vi "PC Engine.vi"(2 "Error In":errorcluster) -> (0 "Error Out":errorcluster, 1 "InvalidResponses":string)   [LabVIEW 2019]
uses:
  State Ctrl (PC).ctl
  <vilib>/NI/STM/TCP/TCP Connection Info.ctl
  <vilib>/NI/STM/SubVIs/MetaDataElement.ctl
  Event Mode.ctl
  PCsend RTrecv CMD.ctl
  <vilib>/NI/STM/TCP/TCP Read Options.ctl
  RT/RTsend PCrecv CMD.ctl
  TypeDef/ConnSettingCluster.ctl
  <vilib>/NI/STM/TCP/Read Meta Data (TCP Ref).vi
  <vilib>/NI/STM/TCP/Read Message (TCP).vi
  <vilib>/NI/STM/TCP/Read Meta Data (TCP Clst).vi
  <vilib>/NI/STM/TCP/Write Message (TCP).vi
  <vilib>/NI/STM/NI STM.lvlib
panel:
  out "Send Conn Info":T1
  in  "State Control":T3
  in  "Recv Port":u16=5555
  in  "Stop":bool
  out "Connected?":bool
  in  "ConnectAttemptLimit":u32=5
  in  "Send Port":u16=5555
  in  "RIO IP Address":string
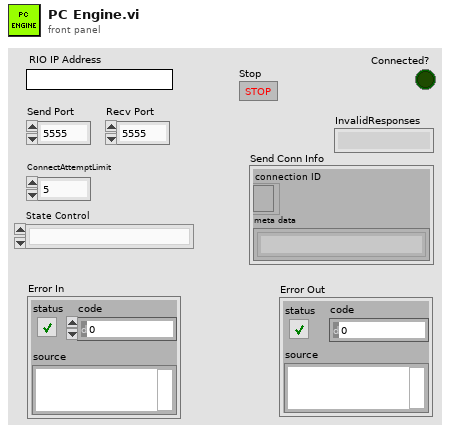
[diagram p1: front panel]
types:
  T1 = typedef "NI STM.lvlib/TCP Connection Info.ctl" = cluster{"connection ID":refnum<k5>, "meta data":T2[]}
  T2 = typedef "NI STM.lvlib/MetaDataElement.ctl" = string
  T3 = typedef "State Ctrl (PC).ctl" = enum16{"", "Send Connect", "Send Connect 2", "Recv Connect", "Recv Connect 2", "No Connection", "Disconnect"}
  T4 = typedef "PCsend RTrecv CMD.ctl" = enum16{"ConnSettings", "Connect", "CMD", "Controller", "PSenable", "ReqCalDate", "Tolerances", "Stable Trigger", "Stop", "VPLimits", "NeedleValve", "SpeedWindow", "FreezeCmdPID", "LoadFPGA", "Tare Pressure"}
  T5 = typedef "Event Mode.ctl" = enum16{"Init", "Get", "Set", "Destroy"}
  T6 = cluster{"Command":string, "Flattened Data":string}
  T7 = typedef "ConnSettingCluster.ctl" = cluster{"ConnectAttemptLimit(5)":u32, "IP Address":string, "Send Port":u16, "Recv Port":u16}
  T8 = typedef "NI STM.lvlib/TCP Read Options.ctl" = cluster{"ignore timeout error":bool, "timeout ms (1000)":i32}
  T9 = typedef "RTsend PCrecv CMD.ctl" = enum16{"Data", "Connected?", "CalFileDate"}
  T10 = cluster{"connection ID":bool, "meta data":bool[]}
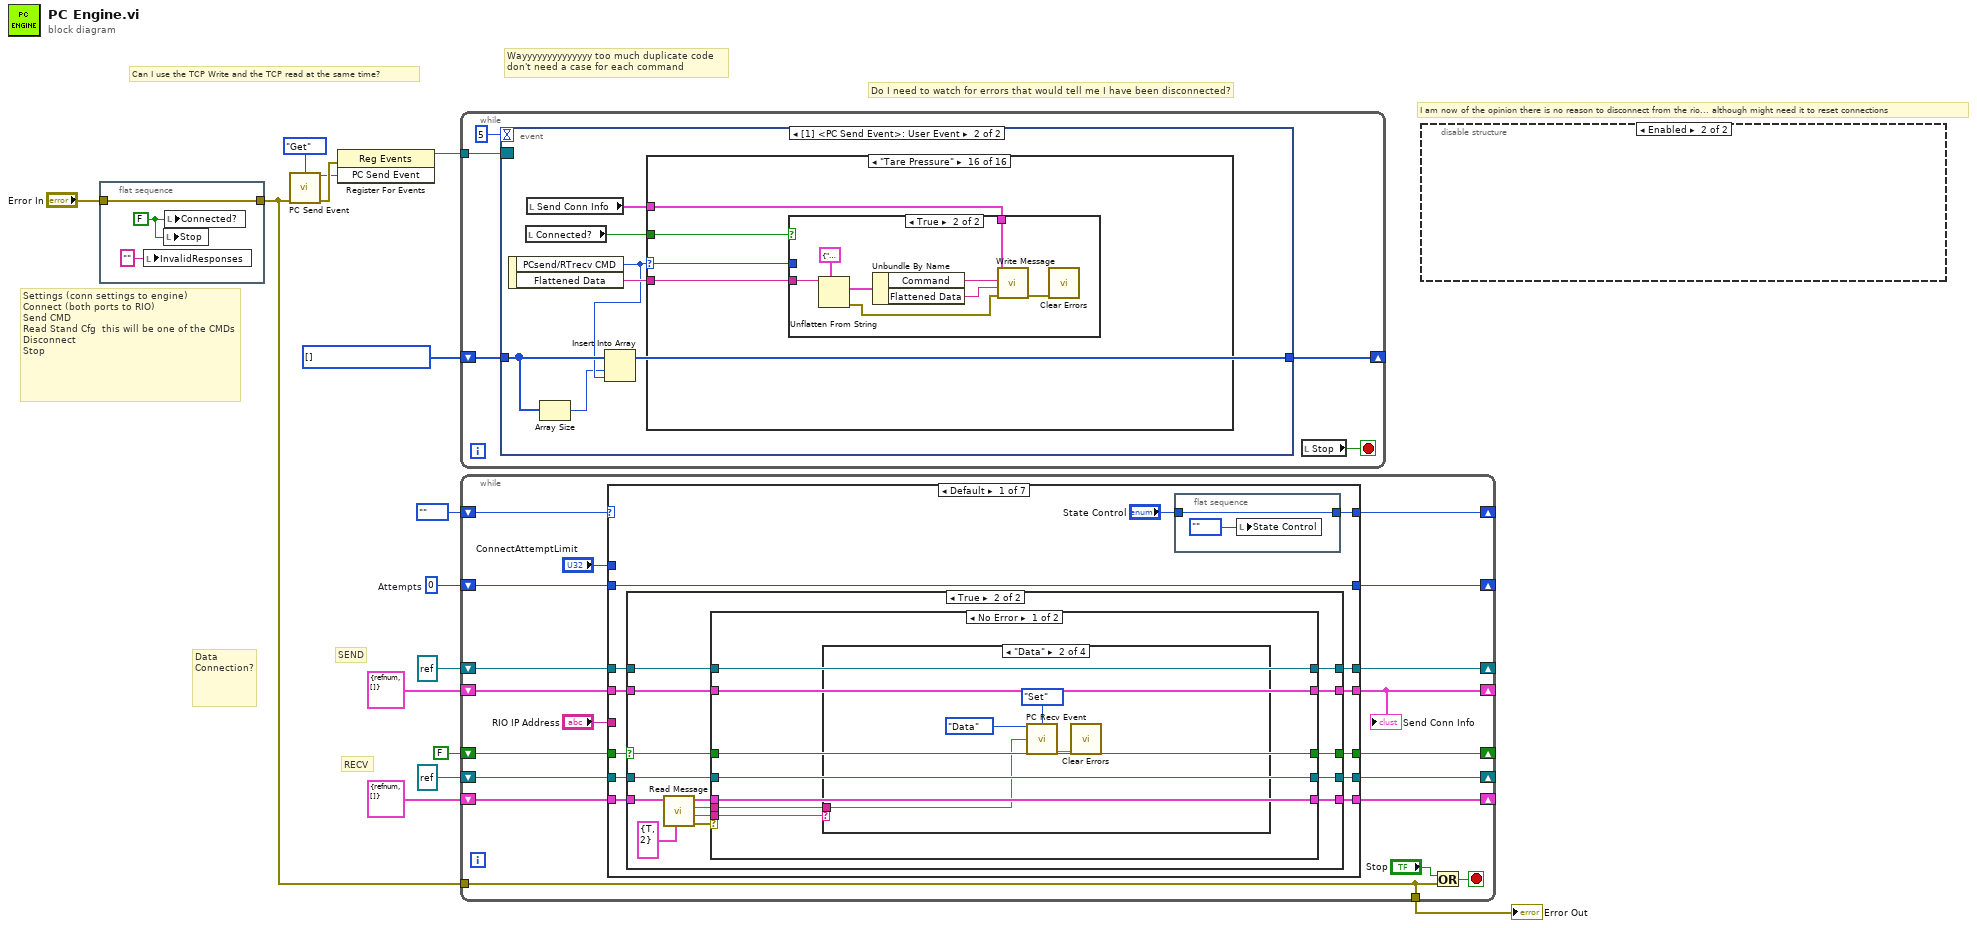
[diagram p0: block diagram]
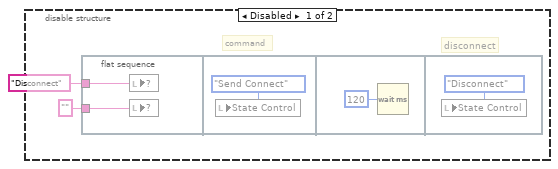
[diagram p2: hidden frame]
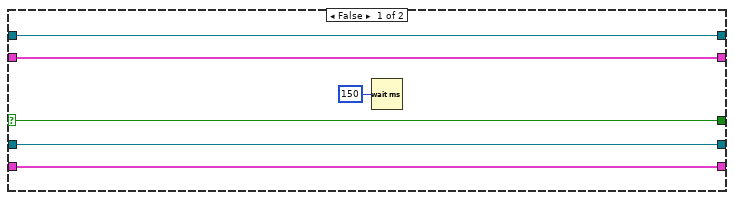
[diagram p3: hidden frame]
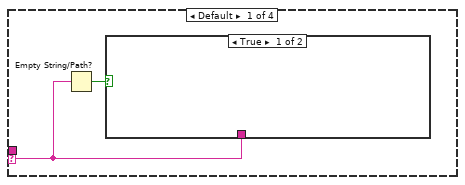
[diagram p4: hidden frame]
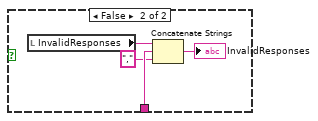
[diagram p5: hidden frame]
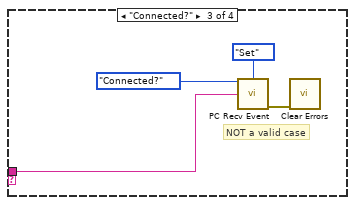
[diagram p6: hidden frame]
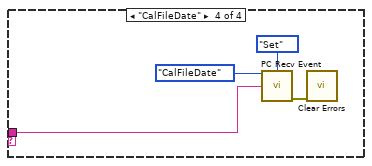
[diagram p7: hidden frame]
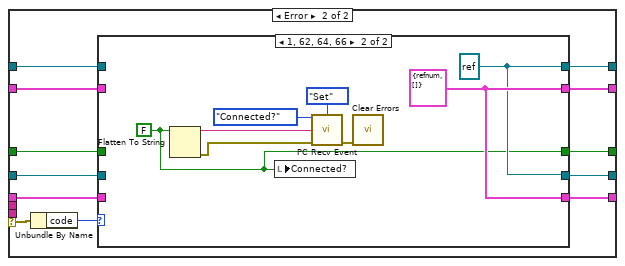
[diagram p8: hidden frame]
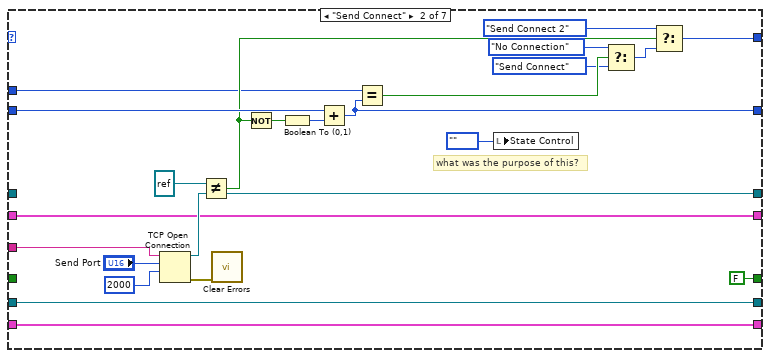
[diagram p10: hidden frame]
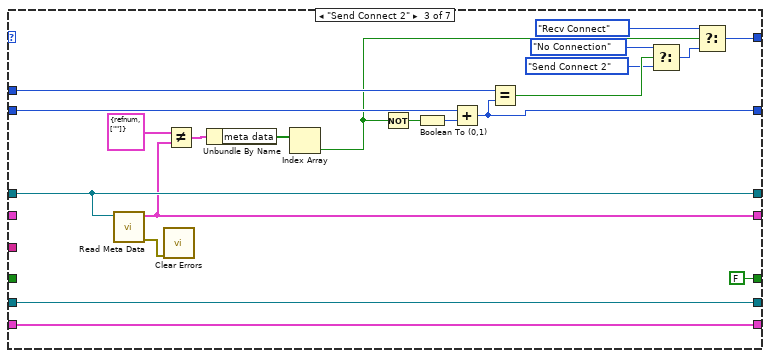
[diagram p11: hidden frame]
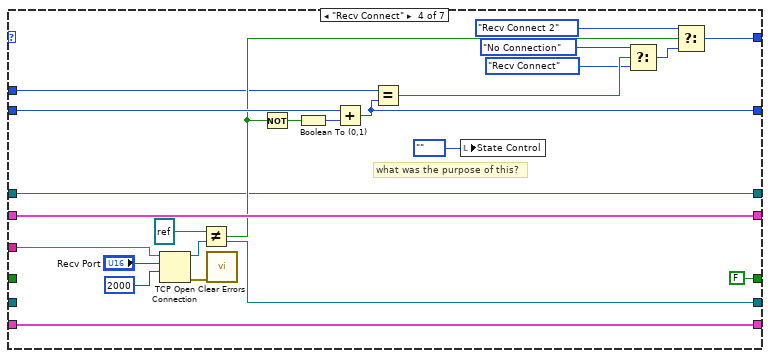
[diagram p12: hidden frame]
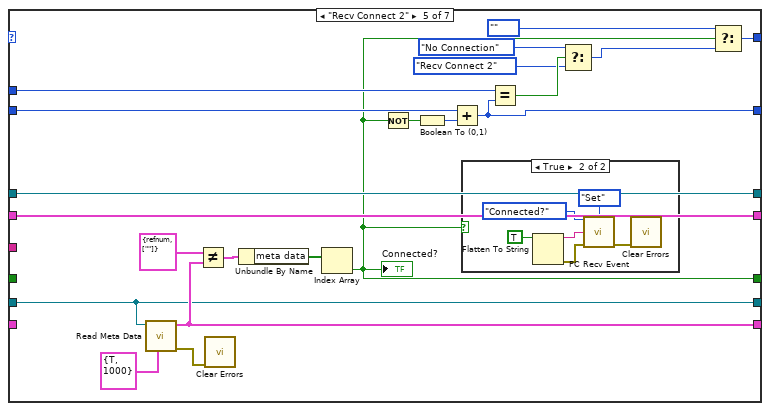
[diagram p13: hidden frame]
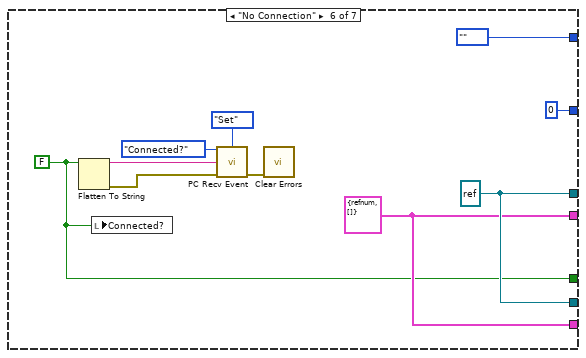
[diagram p15: hidden frame]
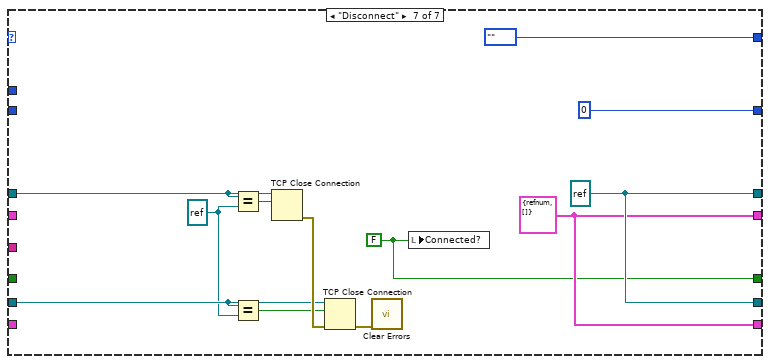
[diagram p16: hidden frame]
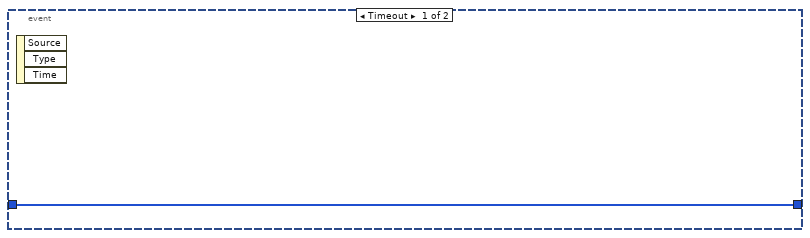
[diagram p17: hidden frame]
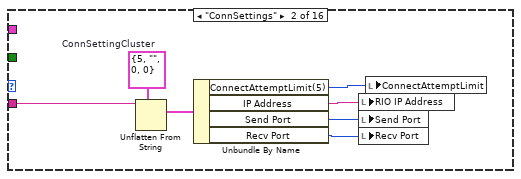
[diagram p19: hidden frame]
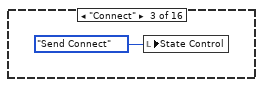
[diagram p20: hidden frame]
diagram:
  w1 = T4[] [] items=["ConnSettings", "Connect", "CMD", "Controller", "PSenable", "ReqCalDate", "Tolerances", "Stable Trigger", "Stop", "VPLimits", "NeedleValve", "SpeedWindow", "FreezeCmdPID", "LoadFPGA", "Tare Pressure"]
  w13 = u32 0  # Attempts
  # "Wayyyyyyyyyyyyyy too much duplicate code\ndon't need a case for each command"
  # "I am now of the opinion there is no reason to disconnect from the rio... although might need it to reset connections"
  # "Do I need to watch for errors that would tell me I have been disconnected?"
  # "RECV"
  # "SEND"
  # "Can I use the TCP Write and the TCP read at the same time?"
  # "Data\nConnection?"
  # "Settings (conn settings to engine)\nConnect (both ports to RIO)\nSend CMD\nRead Stand Cfg  this will be one of the CMDs\nDisconnect\nStop"
  n1 = flat-sequence {
    tunnel: "Error In" -> [w17]
    tunnel: [w17] -> w11
    frame #0 {
      w18 = FALSE ("Connected?")
      n2 = local write "InvalidResponses"("" ("InvalidResponse")) -> ()
      n3 = local write "Stop"(w18) -> ()
      n4 = local write "Connected?"(w18) -> ()
    }
  }
  n5 = call "PC Send Event.vi"("Mode"=Event_Mode."Get", "Error In"=w11) -> ("PC Send Event"=w6:refnum<user-event>, "Error Out"=w8:errorcluster)  [unwired: 12 in]
  n6 = register-events(error in=w8, w6) -> (reference out=w7:refnum<event-registration>)  [unwired: 1 in, 1 out]
  n7 = while {
    tunnel: w7 -> [w21]
    shift-right: [w19] -> _
    shift-left: w1 -> [w20]
    stop <- w23 stop-if-true
    n8 = event shown="[1] <PC Send Event>: User Event" {
      selector: w21 -> [_ _]
      dyn-events: _ -> [_ _]
      timeout: 5 ("evtime") -> [_ _]
      tunnel: w20 -> [w24 w28]
      tunnel: [w24 w25] -> w19
      event Timeout {
        n9 = event-data() -> ()  [unwired: 1 in, 3 out]
      }
      event User Event {
        n10 = event-data() -> ("PCsend/RTrecv CMD"=w27:T4, "Flattened Data"=w31:string)  [unwired: 1 in]
        n11 = local read "Connected?"() -> (w29:bool)
        n12 = local read "Send Conn Info"() -> (w30:T1)
        n13 = Array Size(array=w28) -> (size(s)=w26:i32)
        n14 = Insert Into Array(array=w28, index=w26, new element=w27) -> (w25:T4[])
        n15 = case shown="\"Tare Pressure\"" w27 {
          selector: w27 -> [_ _ _ _ _ _ _ _ _ _ _ _ _ _ _ w162]
          tunnel: w31 -> [_ w33 _ w42 w53 w64 w75 w86 _ w98 w109 w120 w131 w142 w153 w165]
          tunnel: w30 -> [_ _ _ w40 w51 w62 w73 w84 _ w96 w107 w118 w129 w140 w151 w163]
          tunnel: w29 -> [_ _ _ w41 w52 w63 w74 w85 _ w97 w108 w119 w130 w141 w152 w164]
          frame Default {
          }
          frame "ConnSettings" {
            w32 = T7 {"ConnectAttemptLimit(5)"=5, "IP Address"="", "Send Port"=0, "Recv Port"=0}  # ConnSettingCluster
            n16 = Unflatten From String(type=w32, binary string=w33) -> (value=w38:T7)  [unwired: 3 in, 2 out]
            n17 = Unbundle By Name(w38) -> ("ConnectAttemptLimit(5)"=w36:u32, "IP Address"=w35:string, "Send Port"=w37:u16, "Recv Port"=w34:u16)
            n18 = local write "RIO IP Address"(w35) -> ()
            n19 = local write "Send Port"(w37) -> ()
            n20 = local write "Recv Port"(w34) -> ()
            n21 = local write "ConnectAttemptLimit"(w36) -> ()
          }
          frame "Connect" {
            n22 = local write "State Control"(State_Ctrl_(PC)."Send Connect" ("State Control")) -> ()
          }
          frame "CMD" {
            n23 = case shown="True" w41 {
              tunnel: w42 -> [_ w50]
              tunnel: w40 -> [_ w45]
              frame False {
              }
              frame True {
                n24 = Unflatten From String(type=T6 {"Command"="", "Flattened Data"=""} ("cluster"), binary string=w50) -> (value=w49:T6, error out=w43:errorcluster)  [unwired: 3 in, 1 out]
                n25 = Unbundle By Name(w49) -> ("Command"=w46:string, "Flattened Data"=w47:string)
                n26 = call-poly <vilib>:"Write Message.vi"("error in"=w43, "data"=w47, "name"=w46, "connection info in"=w45) -> ("error out"=w44:errorcluster)  [unwired: 6 in, 1 out]
                n27 = call <vilib>:"Clear Errors.vi"("error in (no error)"=w44) -> ()  [unwired: 5 in, 2 out]
              }
            }
          }
          frame "Controller" {
            n28 = case shown="True" w52 {
              tunnel: w53 -> [_ w61]
              tunnel: w51 -> [_ w56]
              frame False {
              }
              frame True {
                n29 = Unflatten From String(type=T6 {"Command"="", "Flattened Data"=""} ("cluster"), binary string=w61) -> (value=w60:T6, error out=w54:errorcluster)  [unwired: 3 in, 1 out]
                n30 = Unbundle By Name(w60) -> ("Command"=w57:string, "Flattened Data"=w58:string)
                n31 = call-poly <vilib>:"Write Message.vi"("error in"=w54, "data"=w58, "name"=w57, "connection info in"=w56) -> ("error out"=w55:errorcluster)  [unwired: 6 in, 1 out]
                n32 = call <vilib>:"Clear Errors.vi"("error in (no error)"=w55) -> ()  [unwired: 5 in, 2 out]
              }
            }
          }
          frame "PSenable" {
            n33 = case shown="True" w63 {
              tunnel: w64 -> [_ w72]
              tunnel: w62 -> [_ w67]
              frame False {
              }
              frame True {
                n34 = Unflatten From String(type=T6 {"Command"="", "Flattened Data"=""} ("cluster"), binary string=w72) -> (value=w71:T6, error out=w65:errorcluster)  [unwired: 3 in, 1 out]
                n35 = Unbundle By Name(w71) -> ("Command"=w68:string, "Flattened Data"=w69:string)
                n36 = call-poly <vilib>:"Write Message.vi"("error in"=w65, "data"=w69, "name"=w68, "connection info in"=w67) -> ("error out"=w66:errorcluster)  [unwired: 6 in, 1 out]
                n37 = call <vilib>:"Clear Errors.vi"("error in (no error)"=w66) -> ()  [unwired: 5 in, 2 out]
              }
            }
          }
          frame "ReqCalDate" {
            n38 = case shown="True" w74 {
              tunnel: w75 -> [_ w83]
              tunnel: w73 -> [_ w78]
              frame False {
              }
              frame True {
                n39 = Unflatten From String(type=T6 {"Command"="", "Flattened Data"=""} ("cluster"), binary string=w83) -> (value=w82:T6, error out=w76:errorcluster)  [unwired: 3 in, 1 out]
                n40 = Unbundle By Name(w82) -> ("Command"=w79:string, "Flattened Data"=w80:string)
                n41 = call-poly <vilib>:"Write Message.vi"("error in"=w76, "data"=w80, "name"=w79, "connection info in"=w78) -> ("error out"=w77:errorcluster)  [unwired: 6 in, 1 out]
                n42 = call <vilib>:"Clear Errors.vi"("error in (no error)"=w77) -> ()  [unwired: 5 in, 2 out]
              }
            }
          }
          frame "Tolerances" {
            n43 = case shown="True" w85 {
              tunnel: w86 -> [_ w94]
              tunnel: w84 -> [_ w89]
              frame False {
              }
              frame True {
                n44 = Unflatten From String(type=T6 {"Command"="", "Flattened Data"=""} ("cluster"), binary string=w94) -> (value=w93:T6, error out=w87:errorcluster)  [unwired: 3 in, 1 out]
                n45 = Unbundle By Name(w93) -> ("Command"=w90:string, "Flattened Data"=w91:string)
                n46 = call-poly <vilib>:"Write Message.vi"("error in"=w87, "data"=w91, "name"=w90, "connection info in"=w89) -> ("error out"=w88:errorcluster)  [unwired: 6 in, 1 out]
                n47 = call <vilib>:"Clear Errors.vi"("error in (no error)"=w88) -> ()  [unwired: 5 in, 2 out]
              }
            }
          }
          frame "Stop" {
            n48 = local write "Stop"(TRUE ("Stop")) -> ()
          }
          frame "VPLimits" {
            n49 = case shown="True" w97 {
              tunnel: w98 -> [_ w106]
              tunnel: w96 -> [_ w101]
              frame False {
              }
              frame True {
                n50 = Unflatten From String(type=T6 {"Command"="", "Flattened Data"=""} ("cluster"), binary string=w106) -> (value=w105:T6, error out=w99:errorcluster)  [unwired: 3 in, 1 out]
                n51 = Unbundle By Name(w105) -> ("Command"=w102:string, "Flattened Data"=w103:string)
                n52 = call-poly <vilib>:"Write Message.vi"("error in"=w99, "data"=w103, "name"=w102, "connection info in"=w101) -> ("error out"=w100:errorcluster)  [unwired: 6 in, 1 out]
                n53 = call <vilib>:"Clear Errors.vi"("error in (no error)"=w100) -> ()  [unwired: 5 in, 2 out]
              }
            }
          }
          frame "NeedleValve" {
            n54 = case shown="True" w108 {
              tunnel: w109 -> [_ w117]
              tunnel: w107 -> [_ w112]
              frame False {
              }
              frame True {
                n55 = Unflatten From String(type=T6 {"Command"="", "Flattened Data"=""} ("cluster"), binary string=w117) -> (value=w116:T6, error out=w110:errorcluster)  [unwired: 3 in, 1 out]
                n56 = Unbundle By Name(w116) -> ("Command"=w113:string, "Flattened Data"=w114:string)
                n57 = call-poly <vilib>:"Write Message.vi"("error in"=w110, "data"=w114, "name"=w113, "connection info in"=w112) -> ("error out"=w111:errorcluster)  [unwired: 6 in, 1 out]
                n58 = call <vilib>:"Clear Errors.vi"("error in (no error)"=w111) -> ()  [unwired: 5 in, 2 out]
              }
            }
          }
          frame "SpeedWindow" {
            n59 = case shown="True" w119 {
              tunnel: w120 -> [_ w128]
              tunnel: w118 -> [_ w123]
              frame False {
              }
              frame True {
                n60 = Unflatten From String(type=T6 {"Command"="", "Flattened Data"=""} ("cluster"), binary string=w128) -> (value=w127:T6, error out=w121:errorcluster)  [unwired: 3 in, 1 out]
                n61 = Unbundle By Name(w127) -> ("Command"=w124:string, "Flattened Data"=w125:string)
                n62 = call-poly <vilib>:"Write Message.vi"("error in"=w121, "data"=w125, "name"=w124, "connection info in"=w123) -> ("error out"=w122:errorcluster)  [unwired: 6 in, 1 out]
                n63 = call <vilib>:"Clear Errors.vi"("error in (no error)"=w122) -> ()  [unwired: 5 in, 2 out]
              }
            }
          }
          frame "FreezeCmdPID" {
            n64 = case shown="True" w130 {
              tunnel: w131 -> [_ w139]
              tunnel: w129 -> [_ w134]
              frame False {
              }
              frame True {
                n65 = Unflatten From String(type=T6 {"Command"="", "Flattened Data"=""} ("cluster"), binary string=w139) -> (value=w138:T6, error out=w132:errorcluster)  [unwired: 3 in, 1 out]
                n66 = Unbundle By Name(w138) -> ("Command"=w135:string, "Flattened Data"=w136:string)
                n67 = call-poly <vilib>:"Write Message.vi"("error in"=w132, "data"=w136, "name"=w135, "connection info in"=w134) -> ("error out"=w133:errorcluster)  [unwired: 6 in, 1 out]
                n68 = call <vilib>:"Clear Errors.vi"("error in (no error)"=w133) -> ()  [unwired: 5 in, 2 out]
              }
            }
          }
          frame "LoadFPGA" {
            n69 = case shown="True" w141 {
              tunnel: w142 -> [_ w150]
              tunnel: w140 -> [_ w145]
              frame False {
              }
              frame True {
                n70 = Unflatten From String(type=T6 {"Command"="", "Flattened Data"=""} ("cluster"), binary string=w150) -> (value=w149:T6, error out=w143:errorcluster)  [unwired: 3 in, 1 out]
                n71 = Unbundle By Name(w149) -> ("Command"=w146:string, "Flattened Data"=w147:string)
                n72 = call-poly <vilib>:"Write Message.vi"("error in"=w143, "data"=w147, "name"=w146, "connection info in"=w145) -> ("error out"=w144:errorcluster)  [unwired: 6 in, 1 out]
                n73 = call <vilib>:"Clear Errors.vi"("error in (no error)"=w144) -> ()  [unwired: 5 in, 2 out]
              }
            }
          }
          frame "Stable Trigger" {
            n74 = case shown="True" w152 {
              tunnel: w153 -> [_ w161]
              tunnel: w151 -> [_ w156]
              frame False {
              }
              frame True {
                n75 = Unflatten From String(type=T6 {"Command"="", "Flattened Data"=""} ("cluster"), binary string=w161) -> (value=w160:T6, error out=w154:errorcluster)  [unwired: 3 in, 1 out]
                n76 = Unbundle By Name(w160) -> ("Command"=w157:string, "Flattened Data"=w158:string)
                n77 = call-poly <vilib>:"Write Message.vi"("error in"=w154, "data"=w158, "name"=w157, "connection info in"=w156) -> ("error out"=w155:errorcluster)  [unwired: 6 in, 1 out]
                n78 = call <vilib>:"Clear Errors.vi"("error in (no error)"=w155) -> ()  [unwired: 5 in, 2 out]
              }
            }
          }
          frame "Tare Pressure" {
            n79 = case shown="True" w164 {
              tunnel: w165 -> [_ w173]
              tunnel: w163 -> [_ w170]
              tunnel: w162 -> [_ _]
              frame False {
              }
              frame True {
                n80 = Unflatten From String(type=T6 {"Command"="", "Flattened Data"=""} ("cluster"), binary string=w173) -> (value=w172:T6, error out=w168:errorcluster)  [unwired: 3 in, 1 out]
                n81 = Unbundle By Name(w172) -> ("Command"=w166:string, "Flattened Data"=w167:string)
                n82 = call-poly <vilib>:"Write Message.vi"("error in"=w168, "data"=w167, "name"=w166, "connection info in"=w170) -> ("error out"=w169:errorcluster)  [unwired: 6 in, 1 out]
                n83 = call <vilib>:"Clear Errors.vi"("error in (no error)"=w169) -> ()  [unwired: 5 in, 2 out]
              }
            }
          }
        }
      }
    }
    n84 = local read "Stop"() -> (w23:bool)
  }
  n85 = while {
    shift-right: [w187] -> _
    shift-left: refnum<k5> refnum ("connection ID") -> [w190]
    shift-right: [w188] -> _
    shift-left: T1 {"connection ID"=refnum, "meta data"=[]} ("connection info out") -> [w189]
    shift-right: [w191] -> _
    shift-left: State_Ctrl_(PC)."" ("State Control") -> [w192]
    shift-right: [w185] -> _
    shift-left: w13 -> [w186]
    tunnel: w11 -> [w174]
    shift-right: [w178] -> _
    shift-left: refnum<k5> refnum ("connection ID") -> [w180]
    shift-right: [w177] -> _
    shift-left: T1 {"connection ID"=refnum, "meta data"=[]} ("connection info out") -> [w179]
    shift-right: [w175] -> _
    shift-left: FALSE -> [w176]
    tunnel: [w174] -> w2
    stop <- w183 stop-if-true
    n86 = case shown="Default" w192 {
      tunnel: [w205 w301 w319 w345 w363 State_Ctrl_(PC)."" ("State Control") State_Ctrl_(PC)."" ("State Control")] -> w191
      tunnel: w190 -> [w200 _ w320 w327 w364 _ w389]
      tunnel: w189 -> [w201 w296 _ w342 w351 _ _]
      tunnel: [w197 w296 w303 w342 w351 w377 w391] -> w188
      tunnel: [w198 w297 w320 w327 w364 w378 w392] -> w187
      tunnel: w186 -> [w193 w295 w315 w341 w359 _ _]
      tunnel: [w193 w291 w314 w337 w358 u32 0 ("Attempts") u32 0 ("Attempts")] -> w185
      tunnel: "ConnectAttemptLimit" -> [_ w288 w312 w334 w356 _ _]
      tunnel: "RIO IP Address" -> [_ w283 _ w329 _ _ _]
      tunnel: w180 -> [w199 w282 w308 _ w350 _ w386]
      tunnel: w179 -> [w202 w281 w307 w325 _ _ _]
      tunnel: [w195 w282 w308 w326 w350 w378 w392] -> w178
      tunnel: [w194 w281 w307 w325 w352 w377 w391] -> w177
      tunnel: w176 -> [w203 _ _ _ _ _ _]
      tunnel: [w196 FALSE ("Meta Element") FALSE ("Meta Element") FALSE ("Meta Element") w347 w376 w384] -> w175
      frame Default {
        n87 = case shown="True" w203 {
          selector: w203 -> [w209 w220]
          tunnel: w202 -> [w207 w225]
          tunnel: w201 -> [w210 w221]
          tunnel: w200 -> [w211 w219]
          tunnel: w199 -> [w208 w222]
          tunnel: [w211 w217] -> w198
          tunnel: [w210 w215] -> w197
          tunnel: [w209 w218] -> w196
          tunnel: [w208 w216] -> w195
          tunnel: [w207 w214] -> w194
          frame False {
            n88 = Wait (ms)(milliseconds to wait=u32 150) -> ()  [unwired: 1 out]
          }
          frame True {
            n89 = call-poly <vilib>:"Read Message.vi"("options"=T8 {"ignore timeout error"=TRUE, "timeout ms (1000)"=2}, "connection info in"=w225) -> ("error out"=w224:errorcluster, "name"=w213:T2, "data string"=w212:string, "connection info out"=w223:T1)  [unwired: 4 in, 2 out]
            n90 = case shown="No Error" w224 {
              selector: w224 -> [_ w263]
              tunnel: w223 -> [w229 w261]
              tunnel: w222 -> [w230 w260]
              tunnel: w221 -> [w232 w258]
              tunnel: w220 -> [w231 w259]
              tunnel: w219 -> [w233 w257]
              tunnel: [w231 w254] -> w218
              tunnel: [w233 w256] -> w217
              tunnel: [w230 w253] -> w216
              tunnel: [w232 w255] -> w215
              tunnel: [w229 w252] -> w214
              tunnel: w213 -> [w228 _]
              tunnel: w212 -> [w227 _]
              frame No Error {
                n91 = case shown="\"Data\"" w228 {
                  selector: w228 -> [w235 _ _ _]
                  tunnel: w227 -> [_ w243 w246 w250]
                  frame Default {
                    n92 = Empty String/Path?(string/path=w235) -> (empty?=w234:bool)
                    n93 = case shown="True" w234 {
                      tunnel: w235 -> [_ w238]
                      frame True {
                      }
                      frame False {
                        n94 = local read "InvalidResponses"() -> (w239:string)
                        n95 = Concatenate Strings(w239, w238, "," ("string")) -> (→"InvalidResponses":string)
                      }
                    }
                  }
                  frame "Data" {
                    n96 = call "PC Recv Event.vi"("RTsend/PCrecv CMD"=RTsend_PCrecv_CMD."Data", "Mode"=Event_Mode."Set", "Flattened Data"=w243) -> ("Error Out"=w241:errorcluster)  [unwired: 11 in, 1 out]
                    n97 = call <vilib>:"Clear Errors.vi"("error in (no error)"=w241) -> ()  [unwired: 5 in, 2 out]
                  }
                  frame "Connected?" {
                    # "NOT a valid case"
                    n98 = call "PC Recv Event.vi"("RTsend/PCrecv CMD"=RTsend_PCrecv_CMD."Connected?", "Mode"=Event_Mode."Set", "Flattened Data"=w246) -> ("Error Out"=w245:errorcluster)  [unwired: 11 in, 1 out]
                    n99 = call <vilib>:"Clear Errors.vi"("error in (no error)"=w245) -> ()  [unwired: 5 in, 2 out]
                  }
                  frame "CalFileDate" {
                    n100 = call "PC Recv Event.vi"("RTsend/PCrecv CMD"=RTsend_PCrecv_CMD."CalFileDate", "Mode"=Event_Mode."Set", "Flattened Data"=w250) -> ("Error Out"=w249:errorcluster)  [unwired: 11 in, 1 out]
                    n101 = call <vilib>:"Clear Errors.vi"("error in (no error)"=w249) -> ()  [unwired: 5 in, 2 out]
                  }
                }
              }
              frame Error {
                n102 = Unbundle By Name(w263) -> ("code"=w262:i32)
                n103 = case shown="1, 62, 64, 66" w262 {
                  tunnel: w261 -> [w264 _]
                  tunnel: w260 -> [w265 _]
                  tunnel: w259 -> [w266 _]
                  tunnel: w258 -> [w267 _]
                  tunnel: w257 -> [w268 _]
                  tunnel: [w268 w275] -> w256
                  tunnel: [w267 w276] -> w255
                  tunnel: [w266 w272] -> w254
                  tunnel: [w265 w275] -> w253
                  tunnel: [w264 w276] -> w252
                  frame Default {
                  }
                  frame 1, 62, 64, 66 {
                    w272 = FALSE ("Connected?")
                    w276 = T1 {"connection ID"=refnum, "meta data"=[]} ("connection info out")
                    w275 = refnum<k5> refnum ("connection ID")
                    n104 = Flatten To String(anything=w272) -> (data string=w273:string, error out=w271:errorcluster)  [unwired: 3 in, 1 out]
                    n105 = local write "Connected?"(w272) -> ()
                    n106 = call "PC Recv Event.vi"("RTsend/PCrecv CMD"=RTsend_PCrecv_CMD."Connected?", "Mode"=Event_Mode."Set", "Flattened Data"=w273, "Error In"=w271) -> ("Error Out"=w270:errorcluster)  [unwired: 10 in, 1 out]
                    n107 = call <vilib>:"Clear Errors.vi"("error in (no error)"=w270) -> ()  [unwired: 5 in, 2 out]
                  }
                }
              }
            }
          }
        }
        n108 = flat-sequence {
          tunnel: "State Control" -> [w278]
          tunnel: [w278] -> w205
          frame #0 {
            n109 = local write "State Control"(State_Ctrl_(PC)."" ("State Control")) -> ()
          }
        }
      }
      frame "Send Connect" {
        # "what was the purpose of this?"
        n110 = TCP Open Connection(address=w283, remote port or service name="Send Port", timeout ms (60000)=2000) -> (connection ID=w297:refnum<k5>, error out=w279:errorcluster)  [unwired: 2 in]
        n111 = Not Equal?(x=refnum<k5> refnum ("connection ID"), y=w297) -> (x != y?=w294:bool)
        n112 = call <vilib>:"Clear Errors.vi"("error in (no error)"=w279) -> ()  [unwired: 5 in, 2 out]
        n113 = Not(x=w294) -> (.not. x?=w293:bool)
        n114 = Boolean To (0,1)(Boolean=w293) -> (0, 1=w292:i16)
        n115 = Add(x=w295, y=w292) -> (x+y=w291:u32)
        n116 = Equal?(x=w288, y=w291) -> (x = y?=w290:bool)
        n117 = local write "State Control"(State_Ctrl_(PC)."" ("State Control")) -> ()
        n118 = Select(t=State_Ctrl_(PC)."No Connection" ("State Control"), s=w290, f=State_Ctrl_(PC)."Send Connect" ("State Control")) -> (s? t:f=w289:T3)
        n119 = Select(t=State_Ctrl_(PC)."Send Connect 2" ("State Control"), s=w294, f=w289) -> (s? t:f=w301:T3)
      }
      frame "Send Connect 2" {
        n120 = call-poly <vilib>:"Read Meta Data.vi"("connection ID"=w320) -> ("error out"=w304:errorcluster, "connection info out"=w303:T1)  [unwired: 8 in, 1 out]
        n121 = call <vilib>:"Clear Errors.vi"("error in (no error)"=w304) -> ()  [unwired: 5 in, 2 out]
        n122 = Not Equal?(x=T1 {"connection ID"=refnum, "meta data"=[""]} ("connection info out"), y=w303) -> (x != y?=w322:T10)
        n123 = Unbundle By Name(w322) -> ("meta data"=w311:bool[])
        n124 = Index Array(array=w311) -> (element=w302:bool)  [unwired: 1 in]
        n125 = Not(x=w302) -> (.not. x?=w317:bool)
        n126 = Boolean To (0,1)(Boolean=w317) -> (0, 1=w316:i16)
        n127 = Add(x=w315, y=w316) -> (x+y=w314:u32)
        n128 = Equal?(x=w312, y=w314) -> (x = y?=w313:bool)
        n129 = Select(t=State_Ctrl_(PC)."No Connection" ("State Control"), s=w313, f=State_Ctrl_(PC)."Send Connect 2" ("State Control")) -> (s? t:f=w318:T3)
        n130 = Select(t=State_Ctrl_(PC)."Recv Connect" ("State Control"), s=w302, f=w318) -> (s? t:f=w319:T3)
      }
      frame "Recv Connect" {
        # "what was the purpose of this?"
        n131 = TCP Open Connection(address=w329, remote port or service name="Recv Port", timeout ms (60000)=2000) -> (connection ID=w326:refnum<k5>, error out=w323:errorcluster)  [unwired: 2 in]
        n132 = Not Equal?(x=refnum<k5> refnum ("connection ID"), y=w326) -> (x != y?=w340:bool)
        n133 = call <vilib>:"Clear Errors.vi"("error in (no error)"=w323) -> ()  [unwired: 5 in, 2 out]
        n134 = Not(x=w340) -> (.not. x?=w339:bool)
        n135 = Boolean To (0,1)(Boolean=w339) -> (0, 1=w338:i16)
        n136 = Add(x=w341, y=w338) -> (x+y=w337:u32)
        n137 = Equal?(x=w334, y=w337) -> (x = y?=w336:bool)
        n138 = local write "State Control"(State_Ctrl_(PC)."" ("State Control")) -> ()
        n139 = Select(t=State_Ctrl_(PC)."No Connection" ("State Control"), s=w336, f=State_Ctrl_(PC)."Recv Connect" ("State Control")) -> (s? t:f=w335:T3)
        n140 = Select(t=State_Ctrl_(PC)."Recv Connect 2" ("State Control"), s=w340, f=w335) -> (s? t:f=w345:T3)
      }
      frame "Recv Connect 2" {
        n141 = call-poly <vilib>:"Read Meta Data.vi"("options"=T8 {"ignore timeout error"=TRUE, "timeout ms (1000)"=1000}, "connection ID"=w350) -> ("error out"=w349:errorcluster, "connection info out"=w352:T1)  [unwired: 7 in, 1 out]
        n142 = Not Equal?(x=T1 {"connection ID"=refnum, "meta data"=[""]} ("connection info out"), y=w352) -> (x != y?=w366:T10)
        n143 = call <vilib>:"Clear Errors.vi"("error in (no error)"=w349) -> ()  [unwired: 5 in, 2 out]
        n144 = Unbundle By Name(w366) -> ("meta data"=w355:bool[])
        n145 = Index Array(array=w355) -> (element=w347:bool)  [unwired: 1 in]
        "Connected?" <- w347
        n146 = Not(x=w347) -> (.not. x?=w361:bool)
        n147 = Boolean To (0,1)(Boolean=w361) -> (0, 1=w360:i16)
        n148 = Add(x=w359, y=w360) -> (x+y=w358:u32)
        n149 = case shown="True" w347 {
          frame False {
          }
          frame True {
            n150 = Flatten To String(anything=TRUE) -> (data string=w370:string, error out=w369:errorcluster)  [unwired: 3 in, 1 out]
            n151 = call "PC Recv Event.vi"("RTsend/PCrecv CMD"=RTsend_PCrecv_CMD."Connected?", "Mode"=Event_Mode."Set", "Flattened Data"=w370, "Error In"=w369) -> ("Error Out"=w368:errorcluster)  [unwired: 10 in, 1 out]
            n152 = call <vilib>:"Clear Errors.vi"("error in (no error)"=w368) -> ()  [unwired: 5 in, 2 out]
          }
        }
        n153 = Equal?(x=w356, y=w358) -> (x = y?=w357:bool)
        n154 = Select(t=State_Ctrl_(PC)."No Connection" ("State Control"), s=w357, f=State_Ctrl_(PC)."Recv Connect 2" ("State Control")) -> (s? t:f=w362:T3)
        n155 = Select(t=State_Ctrl_(PC)."" ("State Control"), s=w347, f=w362) -> (s? t:f=w363:T3)
      }
      frame "No Connection" {
        w376 = FALSE
        w377 = T1 {"connection ID"=refnum, "meta data"=[]} ("connection info out")
        w378 = refnum<k5> refnum ("connection ID")
        n156 = Flatten To String(anything=w376) -> (data string=w380:string, error out=w375:errorcluster)  [unwired: 3 in, 1 out]
        n157 = local write "Connected?"(w376) -> ()
        n158 = call "PC Recv Event.vi"("RTsend/PCrecv CMD"=RTsend_PCrecv_CMD."Connected?", "Mode"=Event_Mode."Set", "Flattened Data"=w380, "Error In"=w375) -> ("Error Out"=w374:errorcluster)  [unwired: 10 in, 1 out]
        n159 = call <vilib>:"Clear Errors.vi"("error in (no error)"=w374) -> ()  [unwired: 5 in, 2 out]
      }
      frame "Disconnect" {
        w384 = FALSE ("Connected?")
        w385 = refnum<k5> refnum ("connection ID")
        w391 = T1 {"connection ID"=refnum, "meta data"=[]} ("connection info out")
        w392 = refnum<k5> refnum ("connection ID")
        n160 = Equal?(x=w389, y=w385) -> (x = y?=w388:bool)
        n161 = Equal?(x=w386, y=w385) -> (x = y?=w387:bool)
        n162 = TCP Close Connection(connection ID=w389, abort (F)=w388) -> (error out=w390:errorcluster)  [unwired: 1 in, 1 out]
        n163 = TCP Close Connection(connection ID=w386, abort (F)=w387, error in (no error)=w390) -> (error out=w383:errorcluster)  [unwired: 1 out]
        n164 = call <vilib>:"Clear Errors.vi"("error in (no error)"=w383) -> ()  [unwired: 5 in, 2 out]
        n165 = local write "Connected?"(w384) -> ()
      }
    }
    "Send Conn Info" <- w188
    n166 = Or(x="Stop", y=w174) -> (x .or. y?=w183:bool)
  }
  "Error Out" <- w2
  n167 = disable-structure shown="Enabled" {
    frame Disabled {
      # "disconnect"
      # "command"
      n168 = flat-sequence {
        tunnel: "" ("Flattened Data") -> [w398]
        tunnel: "Disconnect" ("Command") -> [w397]
        frame #0 {
          n169 = local write item#-1(w397) -> ()
          n170 = local write item#-1(w398) -> ()
        }
        frame #1 {
          n171 = local write "State Control"(State_Ctrl_(PC)."Send Connect" ("State Control")) -> ()
        }
        frame #2 {
          n172 = Wait (ms)(milliseconds to wait=u32 120) -> ()  [unwired: 1 out]
        }
        frame #3 {
          n173 = local write "State Control"(State_Ctrl_(PC)."Disconnect" ("State Control")) -> ()
        }
      }
    }
    frame Enabled {
    }
  }
